vi "Create Named Data Structures.vi"(8 "error in (no error)":errorcluster, 9 "Analog Data":T1, 10 "Analog Data Queue Name":string="Analog Input Data", 11 "Loop Name (DAQ Loop)":string="DAQ Loop") -> (0 "error out":errorcluster, 3 "Named Data Structures":T2)   [LabVIEW 2010, in "Core SubVIs.lvlib"]
doc: "This VI creates the DAQ Loop name and the Analog Data Queue for use throughout the program."
uses:
  Core SubVIs.lvlib
  Controls/TYPE - Named Data Structures.ctl
  Controls/TYPE - Analog Data.ctl
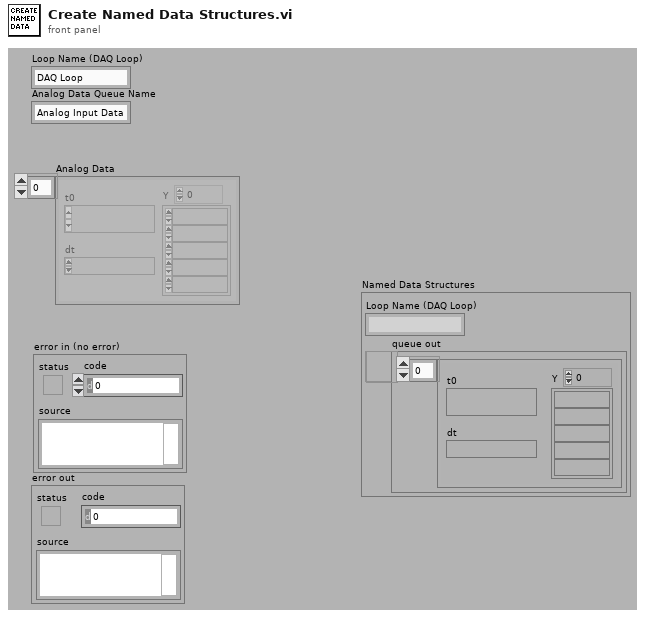
[diagram p1: front panel]
types:
  T1 = typedef "Core SubVIs.lvlib/TYPE - Analog Data.ctl" = waveform(dbl)[]
  T2 = typedef "Core SubVIs.lvlib/TYPE - Named Data Structures.ctl" = cluster{"Loop Name (DAQ Loop)":string, "queue out":refnum<queue>}
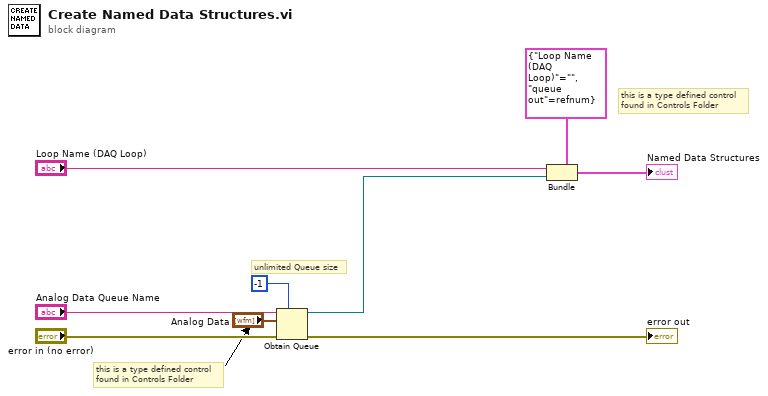
[diagram p0: block diagram]
diagram:
  # "this is a type defined control\nfound in Controls Folder"
  # "this is a type defined control\nfound in Controls Folder"
  # "unlimited Queue size"
  n1 = Obtain Queue(max queue size (-1, unlimited)=-1, name (unnamed)="Analog Data Queue Name", element data type="Analog Data", error in (no error)="error in (no error)") -> (queue out=w2:refnum<queue>, error out=→"error out":errorcluster)  [unwired: 1 in, 1 out]
  n2 = Bundle(cluster=T2 {"Loop Name (DAQ Loop)"="", "queue out"=refnum} ("Named Data Structures"), "Loop Name (DAQ Loop)"="Loop Name (DAQ Loop)", "queue out"=w2) -> (→"Named Data Structures":T2)
